vi "Read Button.vi"(8 "error in (no error)":errorcluster, 11 "ControlMouseDownMsg in":refnum<class "ControlMouseDownMsg.lvclass">) -> (0 "error out":errorcluster, 2 "Button":u16, 3 "ControlMouseDownMsg out":refnum<class "ControlMouseDownMsg.lvclass">)   [LabVIEW 2020, in "MVA Framework.lvlib" / "ActorEvents.lvlib" / "ControlMouseDownMsg.lvclass"]
uses:
  ControlMouseDownMsg.lvclass
  ControlMouseDownMsg.lvclass/ControlMouseDownMsg.ctl
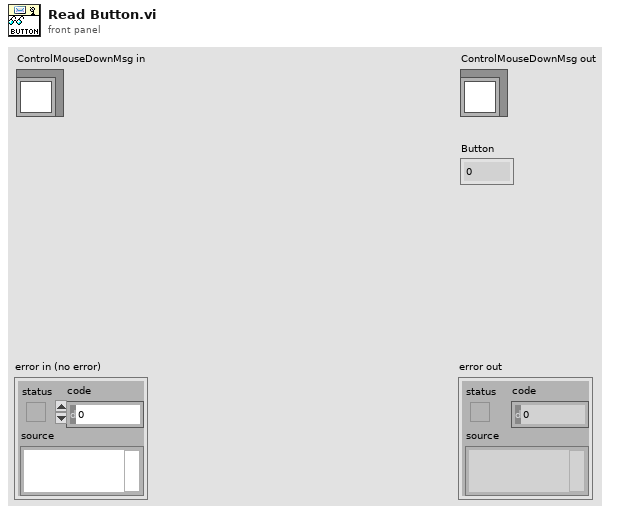
[diagram p1: front panel]
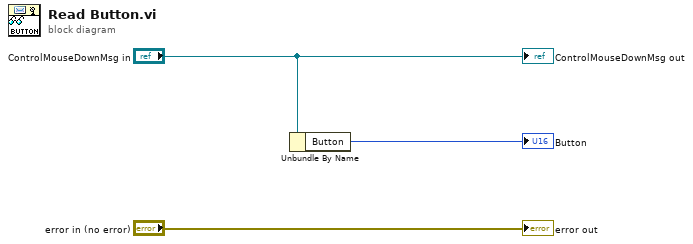
[diagram p0: block diagram]
diagram:
  n1 = Unbundle By Name("ControlMouseDownMsg in") -> ("Button"=→"Button":u16)
  "error out" <- "error in (no error)"
  "ControlMouseDownMsg out" <- "ControlMouseDownMsg in"
